vi "Sample Transfer Container to BlowerHeater.vi"(4 "Container":T2) -> (1 "Blower/Heater":T1)   [LabVIEW 2015, in "cRIO-Carbondioxide.lvlib" / "cRIO-CO2.lvlib" / "cRIO-CO2.lvclass"]
uses:
  cRIO-CO2.lvclass
  Controls/Sample Transfer Container Enumerator.ctl
  Blowers Heaters Enumerator.ctl
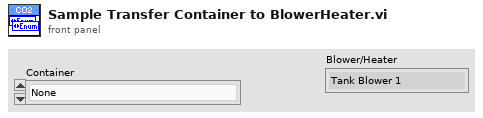
[diagram p1: front panel]
types:
  T1 = typedef "cRIO-Carbondioxide.lvlib/cRIO-CO2.lvlib/cRIO-CO2.lvclass/Blowers Heaters Enumerator.ctl" = enum16{"Tank Blower 1", "Tank Blower 2", "Tank Blower 3", "Tank Blower 4", "Syringe Blower", "Syringe Heater", "Piston Heater", "Undefined"}
  T2 = typedef "Sample Transfer Container Enumerator.ctl" = enum16{"None", "Sample 1", "Sample 2", "Sample 3", "Sample 4", "Sample 5", "Storage 01", "Storage 02", "Storage 03", "Storage 04", "Storage 05", "Storage 06", "Storage 07", "Storage 08", "Storage 09", "Storage 10", "Storage 11", "Storage 12", "Syringe", "Undefined"}
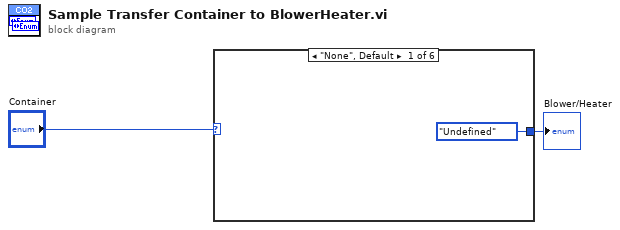
[diagram p0: block diagram]
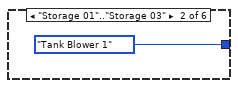
[diagram p2: hidden frame]
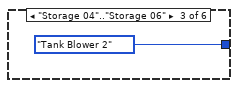
[diagram p3: hidden frame]
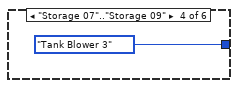
[diagram p4: hidden frame]
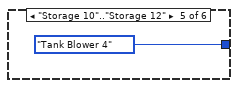
[diagram p5: hidden frame]
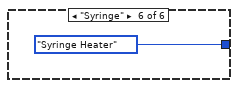
[diagram p6: hidden frame]
diagram:
  n1 = case shown="\"None\", Default" "Container" {
    tunnel: [Blowers_Heaters_Enumerator."Undefined" ("Blower") Blowers_Heaters_Enumerator."Tank Blower 1" ("Blower") Blowers_Heaters_Enumerator."Tank Blower 2" ("Blower") Blowers_Heaters_Enumerator."Tank Blower 3" ("Blower") Blowers_Heaters_Enumerator."Tank Blower 4" ("Blower") Blowers_Heaters_Enumerator."Syringe Heater" ("Blower")] -> w1
    frame "None", Default {
    }
    frame "Storage 01".."Storage 03" {
    }
    frame "Storage 04".."Storage 06" {
    }
    frame "Storage 07".."Storage 09" {
    }
    frame "Storage 10".."Storage 12" {
    }
    frame "Syringe" {
    }
  }
  "Blower/Heater" <- w1
